vi "Convert Cfg Cluster 1 to 2.vi"(11 "Tool Config Cluster_v1":T9={"Tool Type"=0, "Tool SN"=0, "Tool Block"={"Encoder Size"=0, "Encoder Scale"=0, "Encoder Offset"=0, "MaxEncoder"=0, "MinEncoder"=0, "Start Delay"=0.0}, "Motor Block"={"MinMotor Speed"=0, "MaxMotor Speed"=0, "Homing Speed"=90, "Jog Speed"=90, "Inspect Speed"=90, "VBlk Speed"=90, "CleaningPos"=0, "Has Motor"=FALSE, "Use Home Index"=FALSE}, "Verification Block"={"Angle"=90.0, "FlankLength1"=0.0, "FlankLength2"=0.0, "Location"=0.0, "Serial Number"=0}, "Probe Block"={"nProbes"=0, "Probe Param Array"=[]}}) -> (3 "Tool Config Cluster_v2":T1={"Tool Type"=0, "Tool SN"=0, "Tool Block"={"Encoder Size"=0, "Encoder Scale"=0, "Encoder Offset"=0, "MaxEncoder"=0, "MinEncoder"=0, "Start Delay"=0.0}, "Motor Block"={"MinMotor Speed"=0, "MaxMotor Speed"=0, "Homing Speed"=90, "Jog Speed"=90, "Inspect Speed"=90, "VBlk Speed"=90, "CleaningPos"=0, "Safe Zone"=0, "Has Motor"=FALSE, "Use Home Index"=FALSE}, "Verification Block"={"Angle"=90.0, "FlankLength1"=0.0, "FlankLength2"=0.0, "Location"=0.0, "Serial Number"=0}, "Probe Block"={"nProbes"=0, "Probe Param Array"=[]}})   [LabVIEW 2015, in "Tool Cfg.lvlib"]
uses:
  Tool Cfg.lvlib
  _Configuration Cluster_v1--typedef.ctl
  _Tool Block Cluster--typedef.ctl
  _Motor Block Cluster_v1--typedef.ctl
  _Verification Blk Cluster--typedef.ctl
  _Probe Block Cluster--typedef.ctl
  _ProbeConfigParams Cluster--typedef.ctl
  _Sensor Block Cluster--typedef.ctl
  _SensorConfigParams Cluster--typedef.ctl
  _Configuration Cluster_v2--typedef.ctl
  _Motor Block Cluster_v2--typedef.ctl
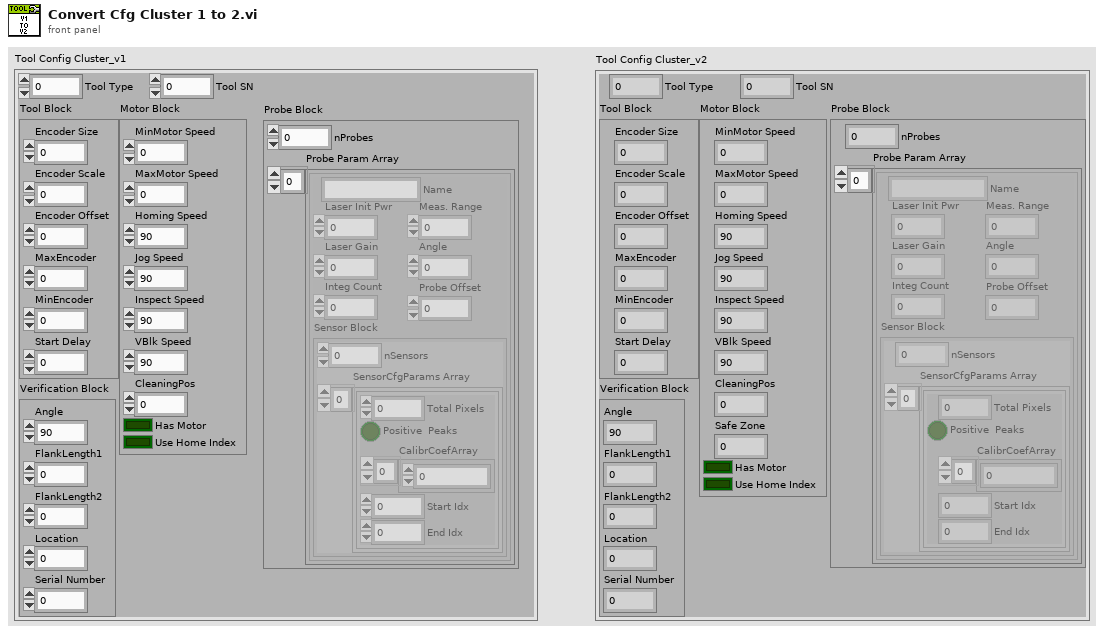
[diagram p1: front panel]
types:
  T1 = typedef "Tool Cfg.lvlib/_Configuration Cluster_v2--typedef.ctl" = cluster{"Tool Type":u16, "Tool SN":u16, "Tool Block":T2, "Motor Block":T3, "Verification Block":T4, "Probe Block":T5}
  T2 = typedef "Tool Cfg.lvlib/_Tool Block Cluster--typedef.ctl" = cluster{"Encoder Size":u16, "Encoder Scale":u32, "Encoder Offset":i32, "MaxEncoder":i32, "MinEncoder":i32, "Start Delay":sgl}
  T3 = typedef "Tool Cfg.lvlib/_Motor Block Cluster_v2--typedef.ctl" = cluster{"MinMotor Speed":u16, "MaxMotor Speed":u16, "Homing Speed":u16, "Jog Speed":u16, "Inspect Speed":u16, "VBlk Speed":u16, "CleaningPos":i32, "Safe Zone":i32, "Has Motor":bool, "Use Home Index":bool}
  T4 = typedef "Tool Cfg.lvlib/_Verification Blk Cluster--typedef.ctl" = cluster{"Angle":sgl, "FlankLength1":sgl, "FlankLength2":sgl, "Location":sgl, "Serial Number":u16}
  T5 = typedef "Tool Cfg.lvlib/_Probe Block Cluster--typedef.ctl" = cluster{"nProbes":u16, "Probe Param Array":T6[]}
  T6 = typedef "Tool Cfg.lvlib/_ProbeConfigParams Cluster--typedef.ctl" = cluster{"Name":string, "Laser Init Pwr":u16, "Laser Gain":u8, "Integ Count":u16, "Meas. Range":sgl, "Angle":sgl, "Probe Offset":sgl, "Sensor Block":T7}
  T7 = typedef "Tool Cfg.lvlib/_Sensor Block Cluster--typedef.ctl" = cluster{"nSensors":u16, "SensorCfgParams Array":T8[]}
  T8 = typedef "Tool Cfg.lvlib/_SensorConfigParams Cluster--typedef.ctl" = cluster{"Total Pixels":u16, "Positive  Peaks":bool, "CalibrCoefArray":dbl[], "Start Idx":u16, "End Idx":u16}
  T9 = typedef "Tool Cfg.lvlib/_Configuration Cluster_v1--typedef.ctl" = cluster{"Tool Type":u16, "Tool SN":u16, "Tool Block":T2, "Motor Block":T10, "Verification Block":T4, "Probe Block":T5}
  T10 = typedef "Tool Cfg.lvlib/_Motor Block Cluster_v1--typedef.ctl" = cluster{"MinMotor Speed":u16, "MaxMotor Speed":u16, "Homing Speed":u16, "Jog Speed":u16, "Inspect Speed":u16, "VBlk Speed":u16, "CleaningPos":i32, "Has Motor":bool, "Use Home Index":bool}
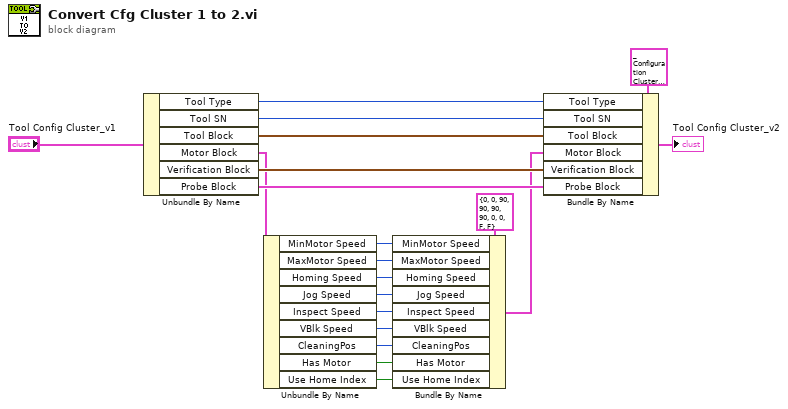
[diagram p0: block diagram]
diagram:
  n1 = Unbundle By Name("Tool Config Cluster_v1") -> ("Tool Type"=w19:u16, "Tool SN"=w18:u16, "Tool Block"=w17:T2, "Motor Block"=w12:T10, "Verification Block"=w16:T4, "Probe Block"=w15:T5)
  n2 = Unbundle By Name(w12) -> ("MinMotor Speed"=w10:u16, "MaxMotor Speed"=w9:u16, "Homing Speed"=w8:u16, "Jog Speed"=w7:u16, "Inspect Speed"=w6:u16, "VBlk Speed"=w5:u16, "CleaningPos"=w4:i32, "Has Motor"=w3:bool, "Use Home Index"=w2:bool)
  n3 = Bundle By Name(cluster=T3 {"MinMotor Speed"=0, "MaxMotor Speed"=0, "Homing Speed"=90, "Jog Speed"=90, "Inspect Speed"=90, "VBlk Speed"=90, "CleaningPos"=0, "Safe Zone"=0, "Has Motor"=FALSE, "Use Home Index"=FALSE} ("_Motor Block Cluster_v2--typedef"), "MinMotor Speed"=w10, "MaxMotor Speed"=w9, "Homing Speed"=w8, "Jog Speed"=w7, "Inspect Speed"=w6, "VBlk Speed"=w5, "CleaningPos"=w4, "Has Motor"=w3, "Use Home Index"=w2) -> (w1:T3)
  n4 = Bundle By Name(cluster=T1 {"Tool Type"=0, "Tool SN"=0, "Tool Block"={"Encoder Size"=0, "Encoder Scale"=0, "Encoder Offset"=0, "MaxEncoder"=0, "MinEncoder"=0, "Start Delay"=0.0}, "Motor Block"={"MinMotor Speed"=0, "MaxMotor Speed"=0, "Homing Speed"=90, "Jog Speed"=90, "Inspect Speed"=90, "VBlk Speed"=90, "CleaningPos"=0, "Safe Zone"=0, "Has Motor"=FALSE, "Use Home Index"=FALSE}, "Verification Block"={"Angle"=90.0, "FlankLength1"=0.0, "FlankLength2"=0.0, "Location"=0.0, "Serial Number"=0}, "Probe Block"={"nProbes"=0, "Probe Param Array"=[]}} ("_Tool Config Cluster_v2--typedef"), "Tool Type"=w19, "Tool SN"=w18, "Tool Block"=w17, "Motor Block"=w1, "Verification Block"=w16, "Probe Block"=w15) -> (→"Tool Config Cluster_v2":T1)
